vi "AcceptLocationDialogue (SubVI).vi"(8 "error in (no error)":errorcluster, 11 "Step name":string) -> (0 "error out":errorcluster, 3 "Accept or Reposition":bool)   [LabVIEW 2016]
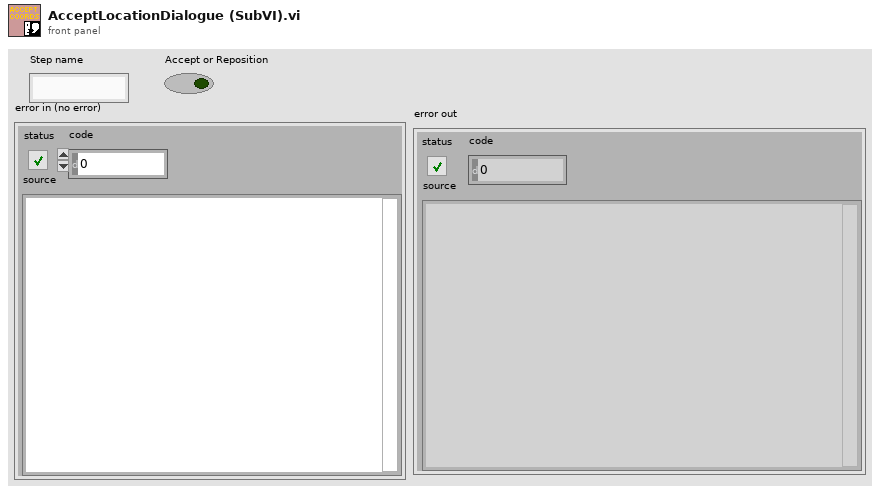
[diagram p1: front panel]
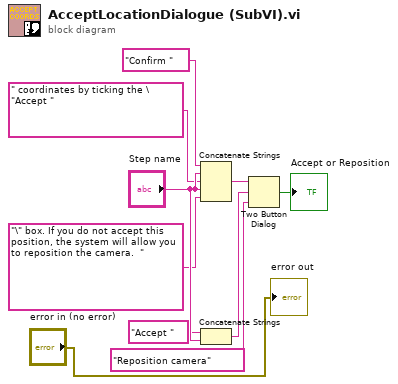
[diagram p0: block diagram]
diagram:
  n1 = Concatenate Strings("Confirm " ("string"), "Step name", " coordinates by ticking the \"Accept " ("string"), "Step name", "\" box. If you do not accept this position, the system will allow you to reposition the camera.  " ("string")) -> (w5:string)
  n2 = Concatenate Strings("Accept " ("string"), "Step name") -> (w3:string)
  n3 = Two Button Dialog(message=w5, 1:"Reposition camera" ("F button name (\"Cancel\")"), 2:w3) -> (T button?=→"Accept or Reposition":bool)
  "error out" <- "error in (no error)"
